vi "Expression Demo.vi"() -> ()   [LabVIEW 2012]
uses:
  calling lua/t_Caching Expression Evaluator Methods.ctl
panel:
  in  "x":string="width*(1+sin(t/2)/3+2*cos(t/5)/3)/2+gauss(noise)"
  in  "y":string="height*(1+cos(t)/3+2*sin(t/3)/3)/2+gauss(noise)"
  out "pict":picture
  in  "noise":dbl(slide) scale=0.0..3.0
  in  "t=":string="t+dt"
  in  "dt":dbl(slide) scale=0.0..0.05
  in  "stop":bool
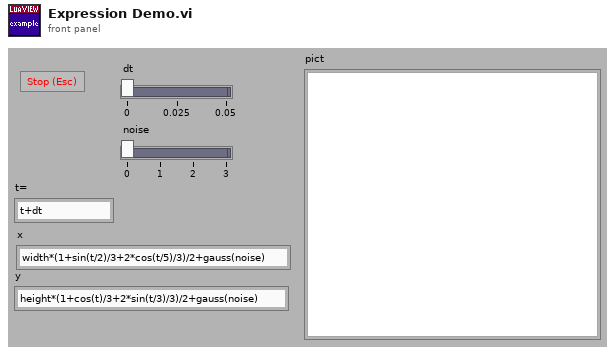
[diagram p1: front panel]
types:
  T1 = typedef "t_Caching Expression Evaluator Methods.ctl" = enum16{"set", "get", "eval", "assign", "execute", "isvalid"}
  T2 = typedef "LVBoundsTypeDef.ctl" = cluster{"Width":u32, "Height":u32}
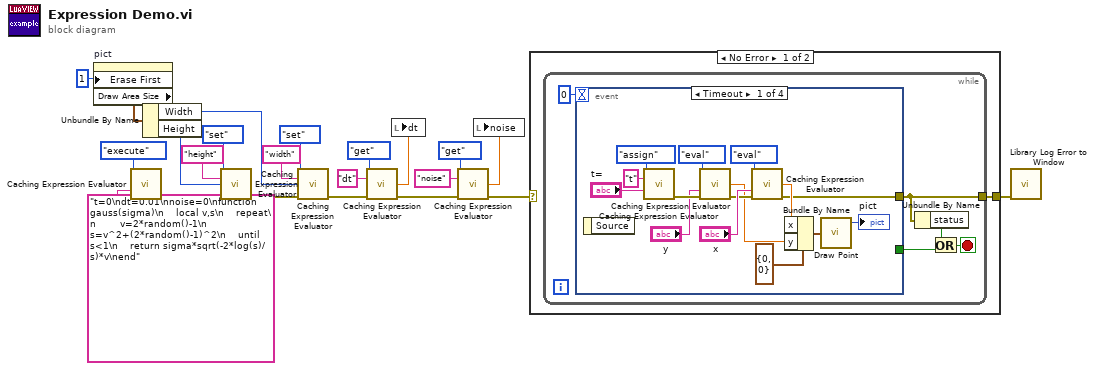
[diagram p0: block diagram]
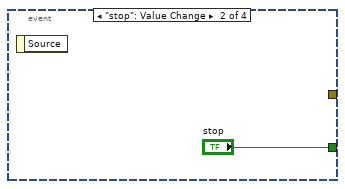
[diagram p2: hidden frame]
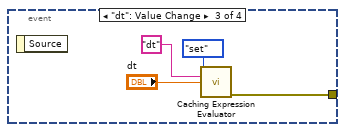
[diagram p3: hidden frame]
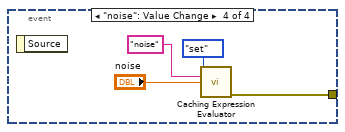
[diagram p4: hidden frame]
diagram:
  n1 = property on="pict" class="Pict"("Erase First"=u8 1) -> ("Draw Area Size"=w6:T2)  [unwired: 2 in, 2 out]
  n2 = call "Caching Expression Evaluator.vi"("method"=t_Caching_Expression_Evaluator_Methods."execute", "expression/scriptlet"="t=0\ndt=0.01\nnoise=0\nfunction gauss(sigma)\n    local v,s\n    repeat\n        v=2*random()-1\n        s=v^2+(2*random()-1)^2\n    until s<1\n    return sigma*sqrt(-2*log(s)/s)*v\nend" ("expression or statements")) -> ("error out"=w10:errorcluster)  [unwired: 12 in, 1 out]
  n3 = Unbundle By Name(w6) -> ("Width"=w2:u32, "Height"=w3:u32)
  n4 = call "Caching Expression Evaluator.vi"("method"=t_Caching_Expression_Evaluator_Methods."set", "variable"="height", "value in"=w3, "error in (no error)"=w10) -> ("error out"=w8:errorcluster)  [unwired: 10 in, 1 out]
  n5 = call "Caching Expression Evaluator.vi"("method"=t_Caching_Expression_Evaluator_Methods."set", "variable"="width", "value in"=w2, "error in (no error)"=w8) -> ("error out"=w7:errorcluster)  [unwired: 10 in, 1 out]
  n6 = call "Caching Expression Evaluator.vi"("method"=t_Caching_Expression_Evaluator_Methods."get", "variable"="dt", "error in (no error)"=w7) -> ("value out"=w16:dbl, "error out"=w12:errorcluster)  [unwired: 11 in]
  n7 = local write "dt"(w16) -> ()
  n8 = call "Caching Expression Evaluator.vi"("method"=t_Caching_Expression_Evaluator_Methods."get", "variable"="noise", "error in (no error)"=w12) -> ("value out"=w15:dbl, "error out"=w21:errorcluster)  [unwired: 11 in]
  n9 = local write "noise"(w15) -> ()
  n10 = case shown="No Error" w21 {
    selector: w21 -> [_ w53]
    tunnel: [w23 w53] -> w22
    frame No Error {
      n11 = while {
        tunnel: [w25] -> w23
        stop <- w27 stop-if-true
        n12 = event shown="[0] Timeout" {
          selector: _ -> [_ _ _ _]
          dyn-events: _ -> [_ _ _ _]
          timeout: 0 -> [_ _ _ _]
          tunnel: [_ "stop" _ _] -> w28
          tunnel: [w29 _ w45 w50] -> w25
          event Timeout {
            n13 = event-data() -> ()  [unwired: 1 in, 1 out]
            n14 = call "Caching Expression Evaluator.vi"("method"=t_Caching_Expression_Evaluator_Methods."assign", "variable"="t", "expression/scriptlet"="t=") -> ("error out"=w39:errorcluster)  [unwired: 11 in, 1 out]
            n15 = call "Caching Expression Evaluator.vi"("method"=t_Caching_Expression_Evaluator_Methods."eval", "expression/scriptlet"="y", "error in (no error)"=w39) -> ("value out"=w31:dbl, "error out"=w35:errorcluster)  [unwired: 11 in]
            n16 = call "Caching Expression Evaluator.vi"("method"=t_Caching_Expression_Evaluator_Methods."eval", "expression/scriptlet"="x", "error in (no error)"=w35) -> ("value out"=w32:dbl, "error out"=w29:errorcluster)  [unwired: 11 in]
            n17 = Bundle By Name(cluster=cluster{"x":i16, "y":i16} {"x"=0, "y"=0} ("point(x,y)"), "x"=w32, "y"=w31) -> (w30:cluster{"x":i16, "y":i16})
            n18 = call <vilib>:"Draw Point.vi"("point(x,y)"=w30) -> ("new picture"=→"pict":picture)  [unwired: 8 in]
          }
          event "stop": Value Change {
            n19 = event-data() -> ()  [unwired: 1 in, 1 out]
          }
          event "dt": Value Change {
            n20 = event-data() -> ()  [unwired: 1 in, 1 out]
            n21 = call "Caching Expression Evaluator.vi"("method"=t_Caching_Expression_Evaluator_Methods."set", "variable"="dt", "value in"="dt") -> ("error out"=w45:errorcluster)  [unwired: 11 in, 1 out]
          }
          event "noise": Value Change {
            n22 = event-data() -> ()  [unwired: 1 in, 1 out]
            n23 = call "Caching Expression Evaluator.vi"("method"=t_Caching_Expression_Evaluator_Methods."set", "variable"="noise", "value in"="noise") -> ("error out"=w50:errorcluster)  [unwired: 11 in, 1 out]
          }
        }
        n24 = Unbundle By Name(w25) -> ("status"=w26:bool)
        n25 = Or(x=w26, y=w28) -> (x .or. y?=w27:bool)
      }
    }
    frame Error {
    }
  }
  n26 = call "Library Log Error to Window.vi"("error in (no error)"=w22) -> ()  [unwired: 13 in, 2 out]
